vi "recuperation_microphones.vi"() -> (3 "Tableau 2":string[](array[string]))   [LabVIEW 2017]
doc: "VI permettant de récupérer la liste des microphones branchés."
panel:
  out "standard output":string
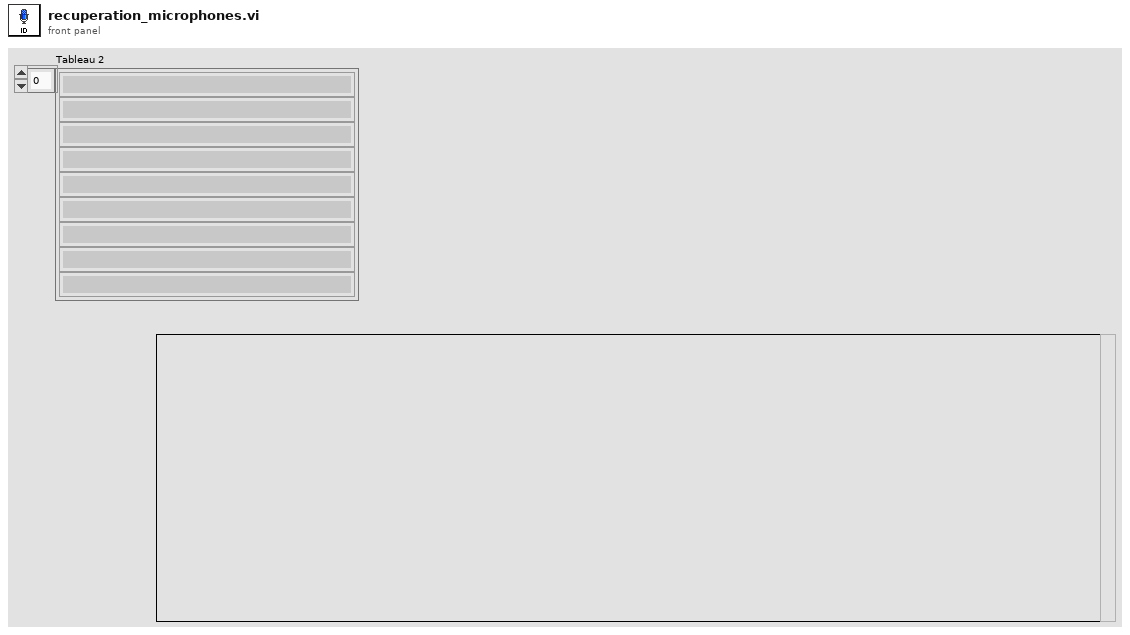
[diagram p1: front panel]
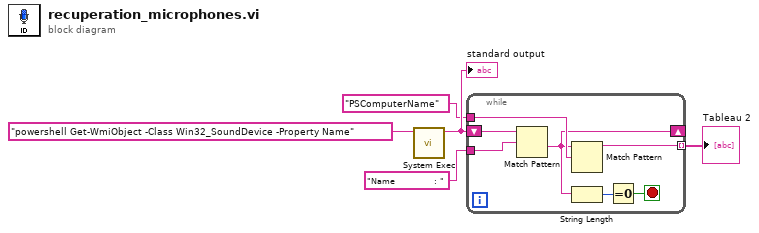
[diagram p0: block diagram]
diagram:
  n1 = call <vilib>:"System Exec.vi"("command line"="powershell Get-WmiObject -Class Win32_SoundDevice -Property Name" ("name or relative path")) -> ("standard output"=w3:string)  [unwired: 7 in, 3 out]
  "standard output" <- w3
  n2 = while {
    shift-right: [w6] -> _
    shift-left: w3 -> [w10]
    tunnel: "Name             : " -> [w9]
    tunnel: [w7] -> w2 mode=indexing
    tunnel: "PSComputerName" ("expression régulière") -> [w8]
    stop <- w11 stop-if-true
    n3 = Match Pattern(string=w10, regular expression=w9) -> (after substring=w6:string)  [unwired: 1 in, 3 out]
    n4 = Match Pattern(string=w6, regular expression=w8) -> (before substring=w7:string)  [unwired: 1 in, 3 out]
    n5 = String Length(string=w6) -> (length=w12:i32)
    n6 = Equal To 0?(x=w12) -> (x = 0?=w11:bool)
  }
  "Tableau 2" <- w2
